vi "NI-DAQmxBaseNew.vi"() -> (0 "error out":errorcluster)   [LabVIEW 2015]
uses:
  Globals/Meas_global.vi
  PWA/PWAtasksGLOBAL.vi
  <vilib>/_DAQmxBase/Internals/DAQmxBase Create Channel (AI-Voltage-Basic).vi
  <vilib>/_DAQmxBase/Internals/DAQmxBase Timing (Sample Clock).vi
  <vilib>/_DAQmxBase/Internals/DAQmxBase Read (Analog 2D DBL NChan NSamp).vi
panel:
  out "AuditTrail":string[](array[string])
  out "input terminal configuration":i32(ring)=10106 items=["default"=-1, "RSE"=10083, "NRSE"=10078, "Differential"=10106, "Pseudodifferential"=12529]
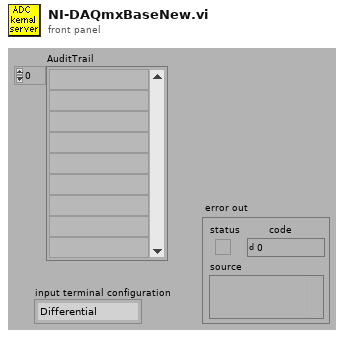
[diagram p1: front panel]
types:
  T1 = typedef "Ch_and_Spans.ctl" = cluster{"high limit (10V)":sgl, "low limit (-10V)":sgl, "Ch No":i16, "Var name":string, "Use Latest Calib":bool}
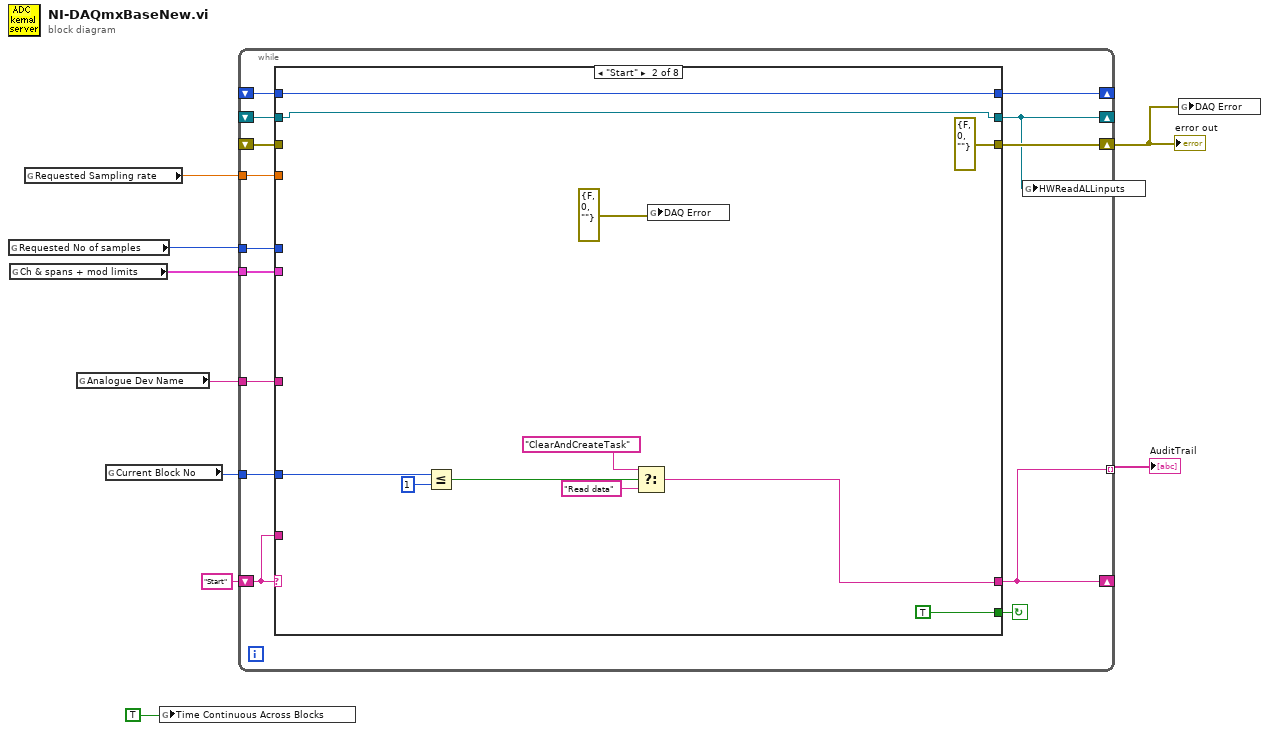
[diagram p0: block diagram]
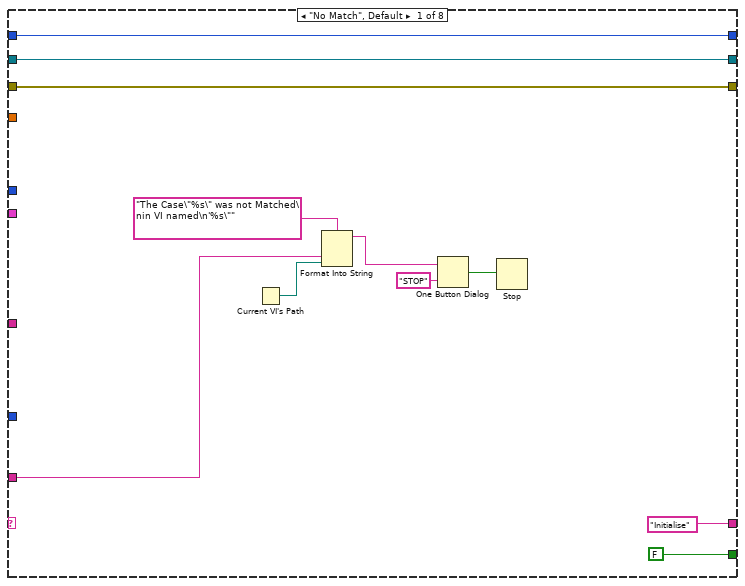
[diagram p2: hidden frame]
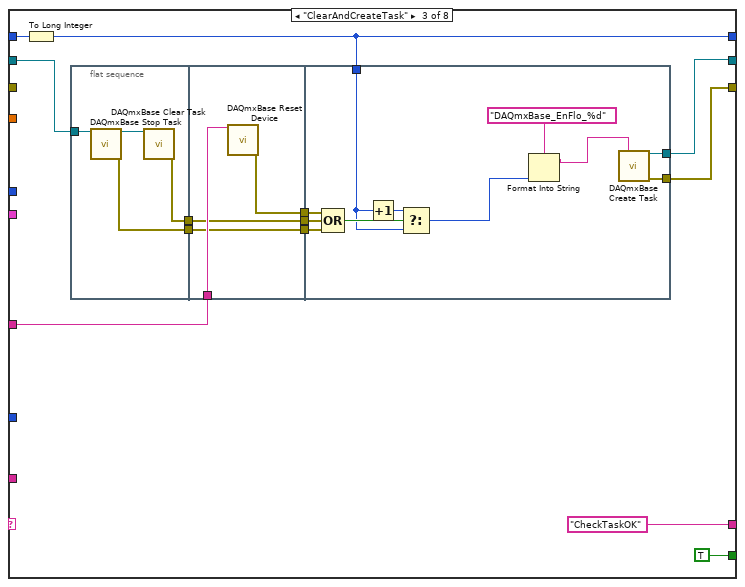
[diagram p3: hidden frame]
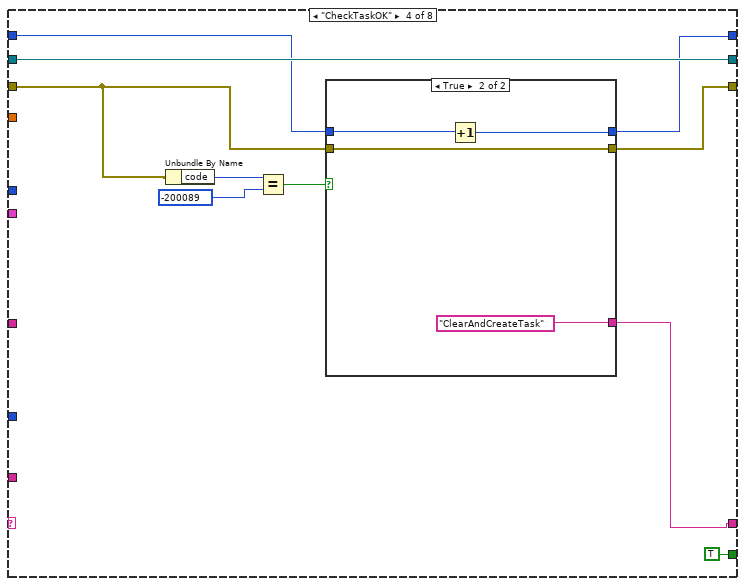
[diagram p4: hidden frame]
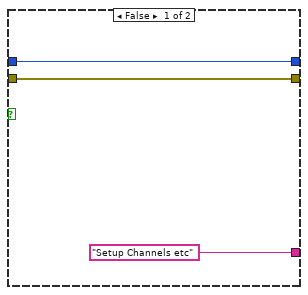
[diagram p5: hidden frame]
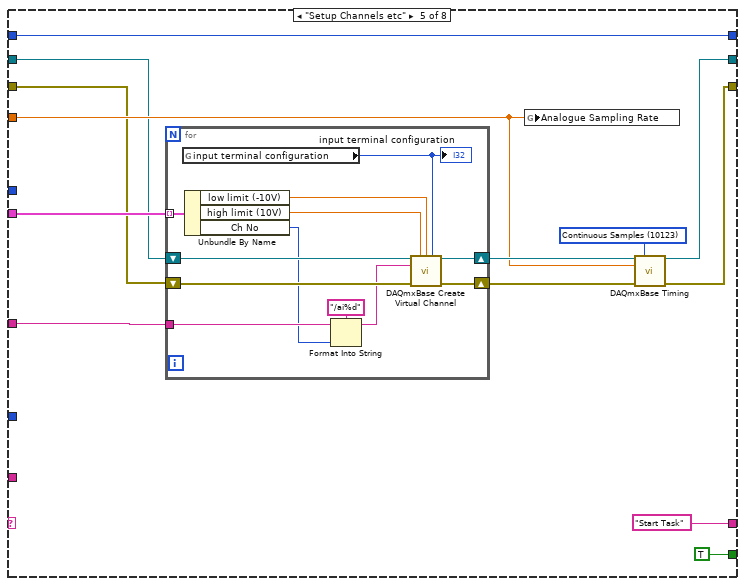
[diagram p6: hidden frame]
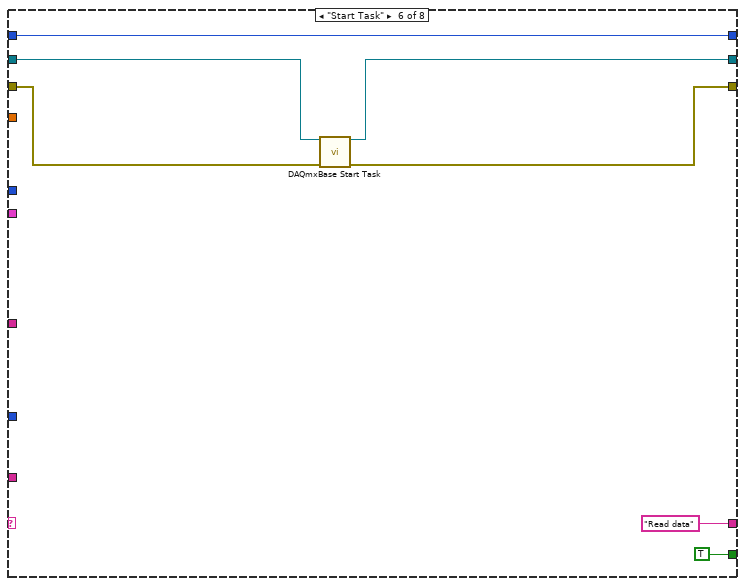
[diagram p7: hidden frame]
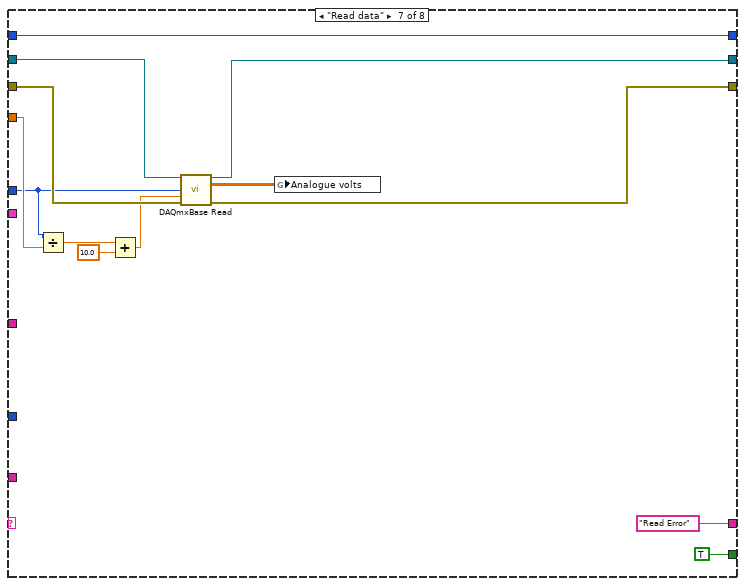
[diagram p8: hidden frame]
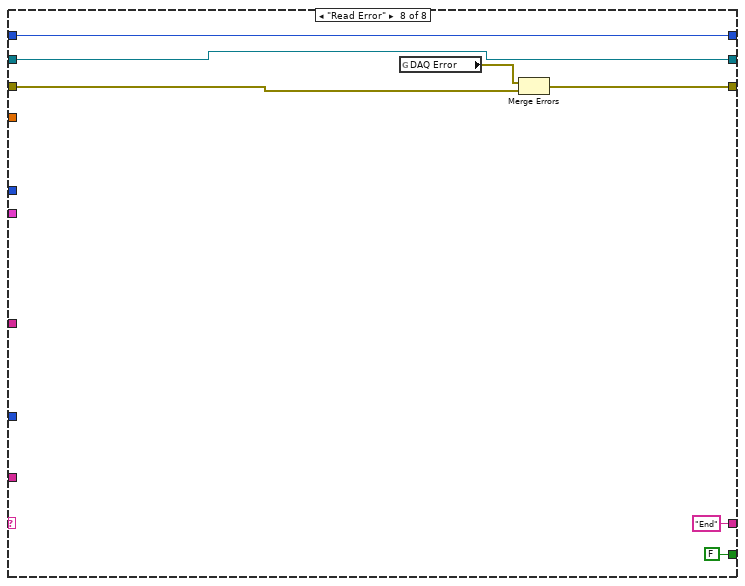
[diagram p9: hidden frame]
diagram:
  n1 = global read "Meas_global.vi" "Requested No of samples"() -> (w2:i32)
  n2 = global read "Meas_global.vi" "Ch & spans + mod limits"() -> (w8:T1[])
  n3 = global read "Meas_global.vi" "Requested Sampling rate"() -> (w5:dbl)
  n4 = global read "PWAtasksGLOBAL.vi" "Analogue Dev Name"() -> (w1:string)
  n5 = global read "Meas_global.vi" "Current Block No"() -> (w7:i32)
  n6 = global write "Meas_global.vi" "Time Continuous Across Blocks"(TRUE ("Time Continuous across Blocks")) -> ()
  n7 = while {
    shift-left: "Start" -> [w22]
    shift-right: [w13] -> _
    shift-right: [w16] -> w6
    shift-left: _ -> [w21]
    tunnel: w5 -> [w20]
    tunnel: w2 -> [w19]
    tunnel: w7 -> [w18]
    tunnel: w8 -> [w17]
    shift-right: [w15] -> _
    shift-left: _ -> [w14]
    tunnel: [w13] -> w4 mode=indexing
    shift-right: [w12] -> _
    shift-left: _ -> [w11]
    tunnel: w1 -> [w10]
    stop <- w23 continue-if-true
    n8 = case shown="\"Start\"" w22 {
      tunnel: [FALSE TRUE TRUE TRUE TRUE TRUE TRUE FALSE] -> w23
      tunnel: ["Initialise" w43 "CheckTaskOK" w82 "Start Task" "Read data" "Read Error" "End" ("f")] -> w13
      tunnel: w22 -> [w29 _ _ _ _ _ _ _]
      tunnel: [w26 errorcluster {"status"=FALSE, "code"=0, "source"=""} ("error out") w46 w79 w103 w123 w127 w144] -> w16
      tunnel: w21 -> [w26 _ _ w78 w95 w122 w139 w145]
      tunnel: w20 -> [_ _ _ _ w100 _ w135 _]
      tunnel: w19 -> [_ _ _ _ _ _ w130 _]
      tunnel: w18 -> [_ w40 _ _ _ _ _ _]
      tunnel: w17 -> [_ _ _ _ w102 _ _ _]
      tunnel: [w25 w42 w52 w84 w99 w124 w136 w143] -> w15
      tunnel: w14 -> [w25 w42 w56 w83 w99 w124 w136 w143]
      tunnel: [w24 w35 w53 w87 w98 w120 w128 w140] -> w12
      tunnel: w11 -> [w24 w35 w55 w87 w97 w121 w129 w140]
      tunnel: w10 -> [_ _ w54 _ w96 _ _ _]
      frame "No Match", Default {
        n9 = Current VI's Path() -> (path=w28:path)
        n10 = Format Into String(format string="The Case\"%s\" was not Matched\nin VI named\n'%s\"" ("Format String"), w29, w28) -> (resulting string=w32:string)  [unwired: 2 in, 1 out]
        n11 = One Button Dialog(message=w32, button name ("OK")="STOP") -> (true=w30:bool)
        n12 = Stop(stop? (T)=w30) -> ()
      }
      frame "Start" {
        n13 = Less Or Equal?(x=w40, y=1) -> (x <= y?=w36:bool)
        n14 = Select(t="ClearAndCreateTask", s=w36, f="Read data") -> (s? t:f=w43:string)
        n15 = global write "Meas_global.vi" "DAQ Error"(errorcluster {"status"=FALSE, "code"=0, "source"=""} ("DAQ Error")) -> ()
      }
      frame "ClearAndCreateTask" {
        n16 = To Long Integer(number=w56) -> (32bit integer=w52:i32)
        n17 = flat-sequence {
          tunnel: w55 -> [w61]
          tunnel: [w60] -> w50
          tunnel: [w59] -> w48
          tunnel: w54 -> [w66]
          tunnel: [w65] -> w51
          tunnel: w50 -> [w65]
          tunnel: [w64] -> w49
          tunnel: w48 -> [w64]
          tunnel: [w63] -> w47
          tunnel: [w77] -> w53
          tunnel: [w76] -> w46
          tunnel: w52 -> [w68]
          tunnel: w51 -> [w71]
          tunnel: w49 -> [w72]
          tunnel: w47 -> [w73]
          frame #0 {
            n18 = call <vilib>:"DAQmxBase Stop Task.vi"("task/channels in"=w61) -> ("task out"=w62:refnum<k21>, "error out"=w60:errorcluster)  [unwired: 13 in]
            n19 = call <vilib>:"DAQmxBase Clear Task.vi"("task in"=w62) -> ("error out"=w59:errorcluster)  [unwired: 14 in]
          }
          frame #1 {
            n20 = call <vilib>:"DAQmxBase Reset Device.vi"("device in"=w66) -> ("error out"=w63:errorcluster)  [unwired: 14 in]
          }
          frame #2 {
            n21 = Compound Arithmetic op=OR(w73, w72, w71) -> (w70:bool)
            n22 = Increment(x=w68) -> (x+1=w69:i32)
            n23 = Select(t=w69, s=w70, f=w68) -> (s? t:f=w67:i32)
            n24 = Format Into String(format string="DAQmxBase_EnFlo_%d" ("new task name"), w67) -> (resulting string=w74:string)  [unwired: 2 in, 1 out]
            n25 = call <vilib>:"DAQmxBase Create Task.vi"("new task name"=w74) -> ("task out"=w77:refnum<k21>, "error out"=w76:errorcluster)  [unwired: 13 in]
          }
        }
      }
      frame "CheckTaskOK" {
        n26 = Unbundle By Name(w78) -> ("code"=w85:i32)
        n27 = Equal?(x=w85, y=-200089 ("code")) -> (x = y?=w80:bool)
        n28 = case shown="True" w80 {
          tunnel: [w90 w93] -> w84
          tunnel: w83 -> [w90 w94]
          tunnel: ["Setup Channels etc" "ClearAndCreateTask"] -> w82
          tunnel: [w88 w91] -> w79
          tunnel: w78 -> [w88 w91]
          frame False {
          }
          frame True {
            n29 = Increment(x=w94) -> (x+1=w93:i32)
          }
        }
      }
      frame "Setup Channels etc" {
        w105 = 10123 items=["Finite Samples"=10178, "Continuous Samples"=10123, "Hardware Timed Single Point"=12522] ("sample mode")
        n30 = for {
          tunnel: w102 -> [w119] mode=indexing
          shift-right: [w117] -> w104
          shift-left: w97 -> [w118]
          shift-right: [w115] -> w106
          shift-left: w95 -> [w116]
          tunnel: w96 -> [w114]
          n31 = global read "Meas_global.vi" "input terminal configuration"() -> (w111:i32)
          "input terminal configuration" <- w111
          n32 = Unbundle By Name(w119) -> ("low limit (-10V)"=w110:sgl, "high limit (10V)"=w109:sgl, "Ch No"=w108:i16)
          n33 = Format Into String(format string="/ai%d", initial string=w114, w108) -> (resulting string=w112:string)  [unwired: 1 in, 1 out]
          n34 = call-poly <vilib>:"DAQmxBase Create Virtual Channel.vi"("task in"=w118, "maximum value"=w109, "minimum value"=w110, "input terminal configuration"=w111, "physical channels"=w112, "error in"=w116) -> ("task out"=w117:refnum<k21>, "error out"=w115:errorcluster)  [unwired: 8 in]
        }
        n35 = global write "Meas_global.vi" "Analogue Sampling Rate"(w100) -> ()
        n36 = call-poly <vilib>:"DAQmxBase Timing.vi"("task/channels in"=w104, "sample mode"=w105, "rate"=w100, "error in"=w106) -> ("task out"=w98:refnum<k21>, "error out"=w103:errorcluster)  [unwired: 10 in]
      }
      frame "Start Task" {
        n37 = call <vilib>:"DAQmxBase Start Task.vi"("task/channels in"=w121, "error in"=w122) -> ("task out"=w120:refnum<k21>, "error out"=w123:errorcluster)  [unwired: 12 in]
      }
      frame "Read data" {
        n38 = Divide(x=w130, y=w135) -> (x/y=w134:dbl)
        n39 = Add(x=w134, y=10.0) -> (x+y=w132:dbl)
        n40 = call-poly <vilib>:"DAQmxBase Read.vi"("task/channels in"=w129, "number of samples per channel"=w130, "timeout"=w132, "error in"=w139) -> ("task out"=w128:refnum<k21>, "data"=w131:dbl[][], "error out"=w127:errorcluster)  [unwired: 9 in]
        n41 = global write "Meas_global.vi" "Analogue volts"(w131) -> ()
      }
      frame "Read Error" {
        n42 = global read "Meas_global.vi" "DAQ Error"() -> (w146:errorcluster)
        n43 = Merge Errors(w146, w145) -> (w144:errorcluster)
      }
    }
    n44 = global write "PWAtasksGLOBAL.vi" "HWReadALLinputs"(w12) -> ()
  }
  "error out" <- w6
  "AuditTrail" <- w4
  n45 = global write "Meas_global.vi" "DAQ Error"(w6) -> ()
